vi "Line Configuration Dialog.vi"(8 "error in":errorcluster, 9 "engine configuration in":refnum<class "engine configuration.lvclass">, 10 "tag bus configurable plugin module configuration":refnum<class "OPC UA Server configuration.lvclass">, 11 "Line":T3 {"OPC UA Data Type" items=["Boolean"=1, "SByte"=2, "Byte"=3, "Int16"=4, "UInt16"=5, "Int32"=6, "UInt32"=7, "Int64"=8, "UInt64"=9, "Float"=10, "Double"=11, "String"=12, "DateTime"=13, "ByteString"=15, "Array of Boolean"=101, "Array of SByte"=102, "Array of Byte"=103, "Array of Int16"=104, "Array of UInt16"=105, "Array of Int32"=106, "Array of UInt32"=107, "Array of Int64"=108, "Array of UInt64"=109, "Array of Float"=110, "Array of Double"=111, "Array of String"=112, "Array of DateTime"=113, "Array of ByteString"=115]}) -> (0 "error out":errorcluster, 1 "success":bool, 2 "changed":bool, 3 "Mappings out":T2 {"Line"."OPC UA Data Type" items=["Boolean"=1, "SByte"=2, "Byte"=3, "Int16"=4, "UInt16"=5, "Int32"=6, "UInt32"=7, "Int64"=8, "UInt64"=9, "Float"=10, "Double"=11, "String"=12, "DateTime"=13, "ByteString"=15, "Array of Boolean"=101, "Array of SByte"=102, "Array of Byte"=103, "Array of Int16"=104, "Array of UInt16"=105, "Array of Int32"=106, "Array of UInt32"=107, "Array of Int64"=108, "Array of UInt64"=109, "Array of Float"=110, "Array of Double"=111, "Array of String"=112, "Array of DateTime"=113, "Array of ByteString"=115]})   [LabVIEW 2013, in "OPC UA Server editor node.lvclass"]
uses:
  OPC UA Server editor node.lvclass
  module/configuration/Line.ctl
  <vilib>/NI/Tag Bus Module Framework/channel/TBM channel.lvclass
  module/configuration/OPC UA Data Type.ctl
  Mappings.ctl
  Map.ctl
  permissions.ctl
  <vilib>/NI/Module Execution Interface/Engine Configuration/engine configuration.lvclass
  module/configuration/OPC UA Server configuration.lvclass
  <vilib>/NI/Tag Bus Module Framework/channel/TBM channel.lvclass/TBM channel.ctl
  <vilib>/NI/Tag Bus/tag/tag descriptor.lvclass/tag descriptor.ctl
  <vilib>/NI/Configuration Framework/serializable configuration/NISE_CEF_serializable configuration.lvclass/NISE_CEF_serializable configuration.ctl
  <vilib>/NI/Tag Bus/tag/write tag name.vi
  <vilib>/NI/Tag Bus/tag/write data type.vi
  <vilib>/NI/Tag Bus Module Framework/channel/Write channel classification.vi
  <vilib>/NI/Tag Bus Module Framework/channel/Read channel classification.vi
  <vilib>/NI/Tag Bus/tag/read data type.vi
  <vilib>/NI/Configuration Framework/serializable configuration/Read UID.vi
  <vilib>/Utility/LVClass/Get LV Class Name.vi
  <vilib>/NI/Configuration Framework/error generator/NISE_error generator.vi
  <vilib>/NI/Tag Bus/tag/tag descriptor.lvclass
panel:
  out "errors":string
  in  "Access Type":T1
  in  "Tag":i32(listbox)
  in  "Data Type":i32(listbox)
  in  "Channel Name":string
  in  "cancel":bool
  in  "ok":bool
  # "#CodeRecommended Add implementation details here. For example, a shared variable URL."
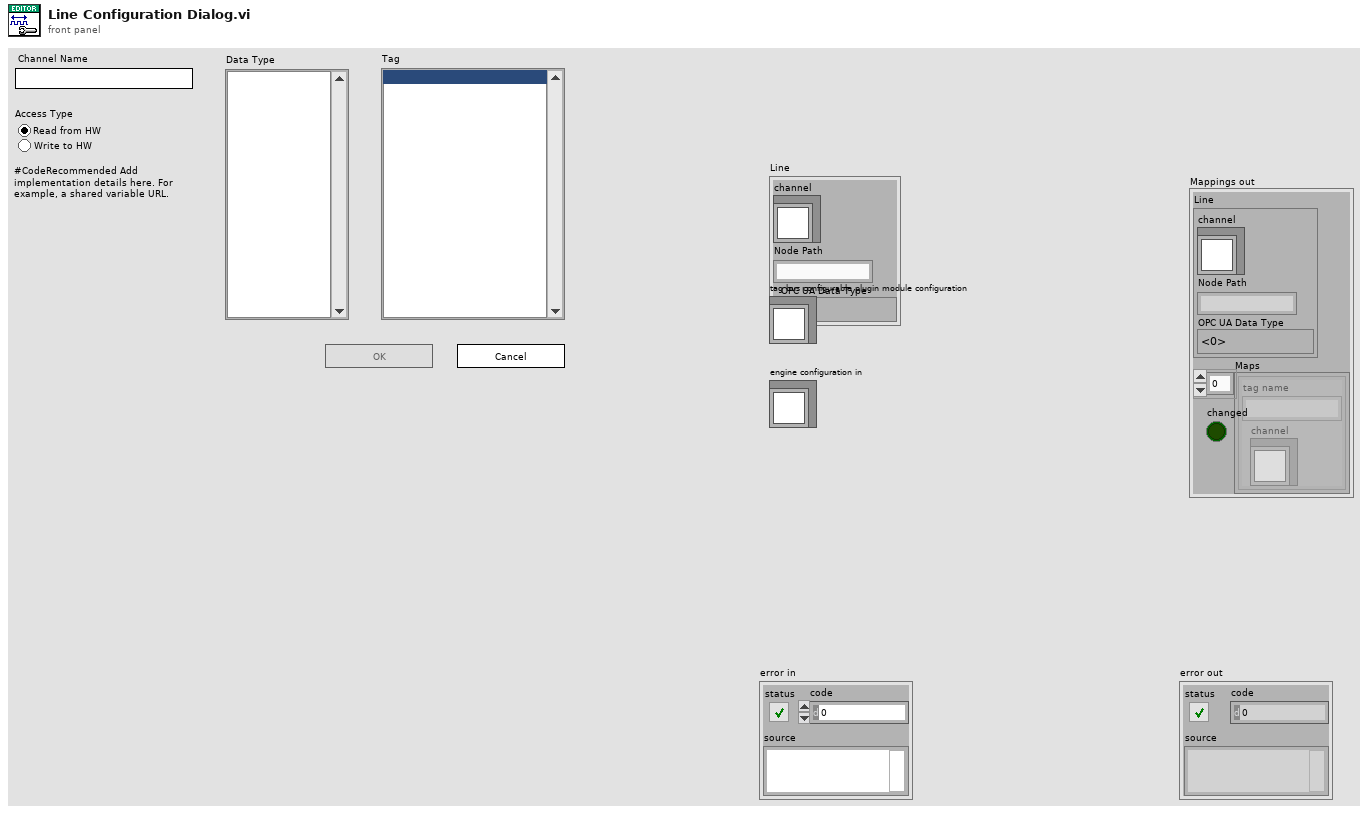
[diagram p1: front panel]
types:
  T1 = typedef "OPC UA Server editor node.lvclass/permissions.ctl" = enum32{"Read from HW", "Write to HW"}
  T2 = typedef "OPC UA Server editor node.lvclass/Mappings.ctl" = cluster{"Line":T3, "Maps":T5[]}
  T3 = typedef "OPC UA Server configuration.lvclass/Line.ctl" = cluster{"channel":refnum<class "TBM channel.lvclass">, "Node Path":string, "OPC UA Data Type":T4}
  T4 = typedef "OPC UA Server configuration.lvclass/OPC UA Data Type.ctl" = u16
  T5 = typedef "OPC UA Server editor node.lvclass/Map.ctl" = cluster{"channel":refnum<class "TBM channel.lvclass">, "tag name":string}
  T6 = typedef "tag bus.lvlib/tag descriptor.lvclass/Data Type.ctl" = enum16{"Double", "Single", "I64", "I32", "I16", "I8", "U64", "U32", "U16", "U8", "Boolean", "String", "Array of Double", "Array of Single", "Array of I64", "Array of I32", "Array of I16", "Array of I8", "Array of U64", "Array of U32", "Array of U16", "Array of U8", "Array of Boolean", "Array of String"}
  T7 = typedef "TBM channel.lvclass/channel classification.ctl" = enum16{"input data", "output data", "processing parameter", "processing result"}
  T8 = enum8{"Enabled", "Disabled", "Disabled and Grayed Out"}
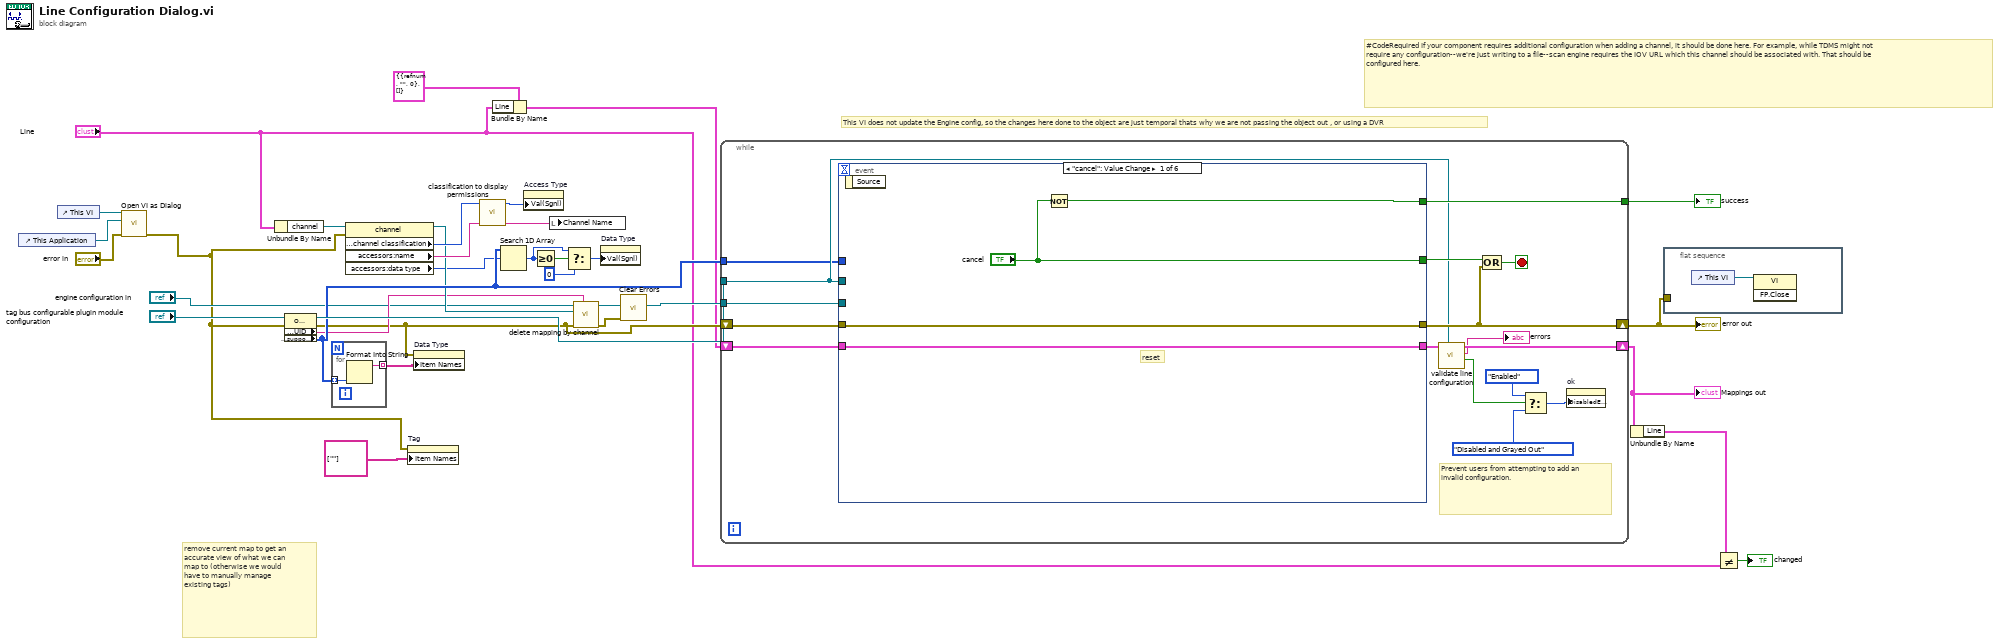
[diagram p0: block diagram]
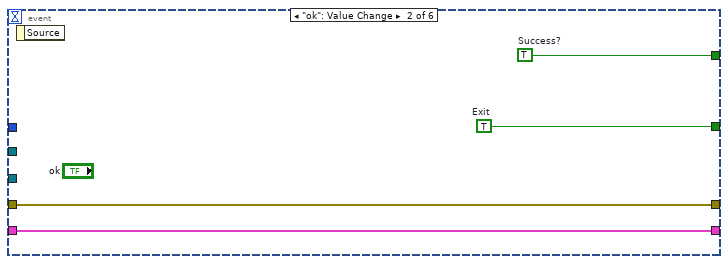
[diagram p2: hidden frame]
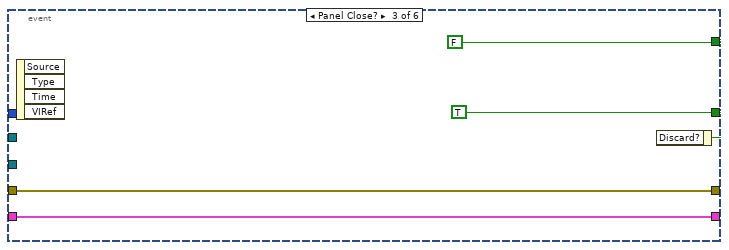
[diagram p3: hidden frame]
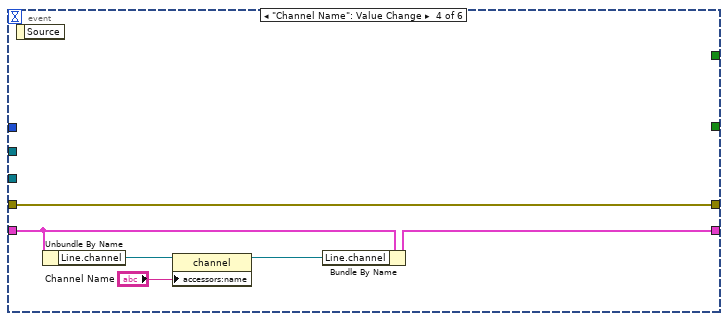
[diagram p4: hidden frame]
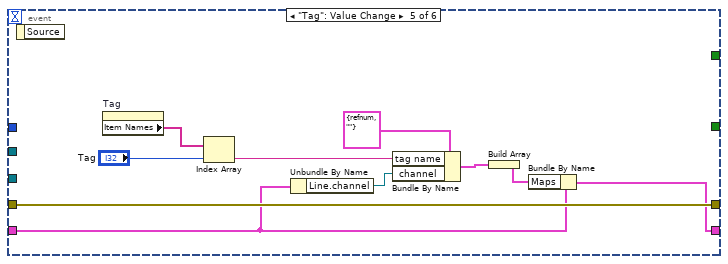
[diagram p5: hidden frame]
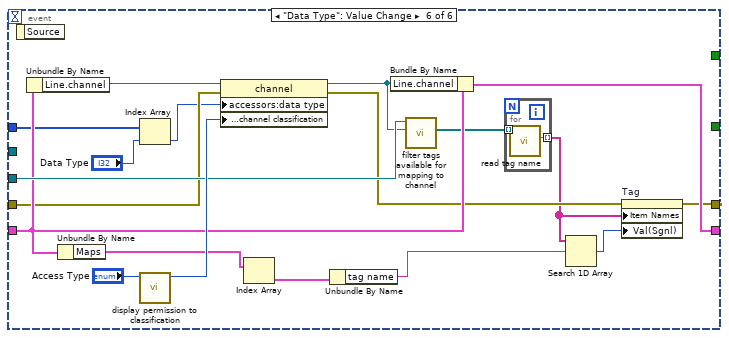
[diagram p6: hidden frame]
diagram:
  # "This VI does not update the Engine config, so the changes here done to the object are just temporal thats why we are not passing the object out , or using a DVR"
  # "remove current map to get an accurate view of what we can map to (otherwise we would have to manually manage existing tags)"
  # "#CodeRequired If your component requires additional configuration when adding a channel, it should be done here. For example, while TDMS might not require any configuration--we're just writing to a file--scan engine requires the IOV URL which this channel should be associated with. That should be configured here."
  n1 = control-ref of="This Application"() -> (w27:refnum<vi>)
  n2 = control-ref of="This VI"() -> (w26:refnum<vi>)
  n3 = call "Open VI as Dialog.vi"("error in (no error)"="error in", "This Application"=w27, "VI in"=w26) -> ("error out"=w6:errorcluster)  [unwired: 8 in]
  n4 = Unbundle By Name("Line") -> ("channel"=w22:refnum<class "TBM channel.lvclass">)
  n5 = property class="OPC UA configuration"(reference="tag bus configurable plugin module configuration", error in=w6) -> (reference out=w29:refnum<class "OPC UA Server configuration.lvclass">, error out=w8:errorcluster, "Properties:UID"=w20:string, "Customize:Properties:supported types"=w28:T6[])
  n6 = for {
    tunnel: w28 -> [w34] mode=indexing
    tunnel: [w33] -> w19 mode=indexing
    n7 = Format Into String(w34) -> (resulting string=w33:string)  [unwired: 3 in, 1 out]
  }
  n8 = property class="channel"(reference=w22, error in=w6) -> (reference out=w21:refnum<class "TBM channel.lvclass">, "data access:channel classification"=w24:T7, "accessors:name"=w23:string, "accessors:data type"=w12:T6)  [unwired: 1 out]
  n9 = property on="Tag" class="LstBox (strict)"(error in=w6, "Item Names"=string[] [""]) -> ()  [unwired: 1 in, 2 out]
  n10 = property on="Data Type" class="LstBox (strict)"(error in=w8, "Item Names"=w19) -> ()  [unwired: 1 in, 2 out]
  n11 = call "classification to display permissions.vi"("channel classification"=w24) -> ("permissions"=w13:T1)  [unwired: 10 in]
  n12 = Bundle By Name(cluster=T2 {"Line"={"channel"=refnum, "Node Path"="", "OPC UA Data Type"=0}, "Maps"=[]} ("Mappings out"), "Line"="Line") -> (w3:T2)
  n13 = Search 1D Array(1D array=w28, element=w12) -> (index of element=w17:i32)  [unwired: 1 in]
  n14 = property on="Access Type" class="RadioBtnsControl (strict)"("Val(Sgnl)"=w13) -> ()  [unwired: 2 in, 2 out]
  n15 = Greater Or Equal To 0?(x=w17) -> (x >= 0?=w18:bool)
  n16 = local write "Channel Name"(w23) -> ()
  n17 = Select(t=w17, s=w18, f=0) -> (s? t:f=w15:i32)
  n18 = call <vilib>:"delete mapping by channel.vi"("owner ID"=w20, "error in"=w8, "channel"=w21, "engine configuration in"="engine configuration in") -> ("error out"=w11:errorcluster, "engine configuration out"=w30:refnum<class "engine configuration.lvclass">)  [unwired: 6 in]
  n19 = property on="Data Type" class="LstBox (strict)"("Val(Sgnl)"=w15) -> ()  [unwired: 2 in, 2 out]
  n20 = call <vilib>:"Clear Errors.vi"("error in (no error)"=w11) -> ()  [unwired: 6 in, 1 out]
  n21 = while {
    shift-right: [w42] -> w25
    shift-left: w8 -> [w49]
    tunnel: [w48] -> w32
    shift-right: [w43] -> w1
    shift-left: w3 -> [w45]
    tunnel: w30 -> [w50]
    tunnel: w29 -> [w37]
    tunnel: w28 -> [w36]
    stop <- w46 stop-if-true
    # "Prevent users from attempting to add an invalid configuration."
    n22 = event shown="[0] \"cancel\": Value Change" {
      selector: _ -> [_ _ _ _ _ _]
      dyn-events: _ -> [_ _ _ _ _ _]
      timeout: _ -> [_ _ _ _ _ _]
      tunnel: w50 -> [_ _ _ _ _ w95]
      tunnel: w49 -> [w54 w58 w62 w68 w78 w89]
      tunnel: [w54 w58 w62 w68 w78 w84] -> w42
      tunnel: [w53 w55 FALSE _ _ _] -> w48
      tunnel: ["cancel" w56 w60 _ _ _] -> w47
      tunnel: w45 -> [w51 w57 w59 w66 w72 w93]
      tunnel: [w51 w57 w59 w67 w69 w92] -> w44
      tunnel: w37 -> [_ _ _ _ _ _]
      tunnel: w36 -> [_ _ _ _ _ w88]
      event "cancel": Value Change {
        # "reset"
        n23 = event-data() -> ()  [unwired: 1 in, 1 out]
        n24 = Not(x="cancel") -> (.not. x?=w53:bool)
      }
      event "ok": Value Change {
        w55 = TRUE  # Success?
        w56 = TRUE  # Exit
        n25 = event-data() -> ()  [unwired: 1 in, 1 out]
      }
      event Panel Close? {
        w60 = TRUE ("cancel")
        n26 = event-data() -> ()  [unwired: 1 in, 4 out]
        n27 = event-data("Discard?"=w60) -> ()  [unwired: 1 in, 1 out]
      }
      event "Channel Name": Value Change {
        n28 = event-data() -> ()  [unwired: 1 in, 1 out]
        n29 = Unbundle By Name(w66) -> ("Line.channel"=w65:refnum<class "TBM channel.lvclass">)
        n30 = property class="channel"(reference=w65, "accessors:name"="Channel Name") -> (reference out=w64:refnum<class "TBM channel.lvclass">)  [unwired: 1 in, 1 out]
        n31 = Bundle By Name(cluster=w66, "Line.channel"=w64) -> (w67:T2)
      }
      event "Tag": Value Change {
        n32 = event-data() -> ()  [unwired: 1 in, 1 out]
        n33 = property on="Tag" class="LstBox (strict)"() -> ("Item Names"=w76:string[])  [unwired: 2 in, 2 out]
        n34 = Index Array(array=w76, index="Tag") -> (element=w75:string)
        n35 = Unbundle By Name(w72) -> ("Line.channel"=w73:refnum<class "TBM channel.lvclass">)
        n36 = Bundle By Name(cluster=T5 {"channel"=refnum, "tag name"=""} ("Map"), "tag name"=w75, "channel"=w73) -> (w71:T5)
        n37 = Build Array(w71) -> (w70:T5[])
        n38 = Bundle By Name(cluster=w72, "Maps"=w70) -> (w69:T2)
      }
      event "Data Type": Value Change {
        n39 = event-data() -> ()  [unwired: 1 in, 1 out]
        n40 = Unbundle By Name(w93) -> ("Line.channel"=w97:refnum<class "TBM channel.lvclass">)
        n41 = Unbundle By Name(w93) -> ("Maps"=w81:T5[])
        n42 = Index Array(array=w88, index="Data Type") -> (element=w86:T6)
        n43 = call "display permission to classification.vi"("display permissions"="Access Type") -> ("channel classification"=w96:T7)  [unwired: 10 in]
        n44 = property class="channel"(reference=w97, error in=w89, "accessors:data type"=w86, "data access:channel classification"=w96) -> (reference out=w94:refnum<class "TBM channel.lvclass">, error out=w85:errorcluster)
        n45 = Index Array(array=w81) -> (element=w80:T5)  [unwired: 1 in]
        n46 = Unbundle By Name(w80) -> ("tag name"=w79:string)
        n47 = Bundle By Name(cluster=w93, "Line.channel"=w94) -> (w92:T2)
        n48 = call <vilib>:"filter tags available for mapping to channel.vi"("channel to map to"=w94, "engine configuration in"=w95) -> ("filtered tags"=w91:refnum<class "tag descriptor.lvclass">[])  [unwired: 8 in, 1 out]
        n49 = for {
          tunnel: w91 -> [w99] mode=indexing
          tunnel: [w98] -> w83 mode=indexing
          n50 = call <vilib>:"read tag name.vi"("system tag in"=w99) -> ("name"=w98:string)  [unwired: 8 in, 2 out]
        }
        n51 = Search 1D Array(1D array=w83, element=w79) -> (index of element=w82:i32)  [unwired: 1 in]
        n52 = property on="Tag" class="LstBox (strict)"(error in=w85, "Item Names"=w83, "Val(Sgnl)"=w82) -> (error out=w84:errorcluster)  [unwired: 1 in, 1 out]
      }
    }
    n53 = call "validate line configuration.vi"("module"=w37, "Mappings in"=w44) -> ("valid?"=w41:bool, "errors"=→"errors":string, "Mappings out"=w43:T2)  [unwired: 7 in]
    n54 = Compound Arithmetic op=OR(w47, w42) -> (w46:bool)
    n55 = Select(t=T8."Enabled" ("Disabled"), s=w41, f=T8."Disabled and Grayed Out") -> (s? t:f=w38:T8)
    n56 = property on="ok" class="Bool"("DisabledEnum"=w38) -> ()  [unwired: 2 in, 2 out]
  }
  "error out" <- w25
  "success" <- w32
  "Mappings out" <- w1
  n57 = Unbundle By Name(w1) -> ("Line"=w2:T3)
  n58 = flat-sequence {
    tunnel: w25 -> [_]
    frame #0 {
      n59 = control-ref of="This VI"() -> (w100:refnum<vi>)
      n60 = invoke class="VI" method="FP.Close"(reference=w100) -> ()  [unwired: 2 in, 3 out]
    }
  }
  n61 = Not Equal?(x=w2, y="Line") -> (x != y?=→"changed":bool)
